vi "Boolean Latch.vi"(1 "Input":bool) -> (0 "Output":bool)   [LabVIEW 2011]
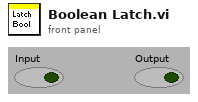
[diagram p1: front panel]
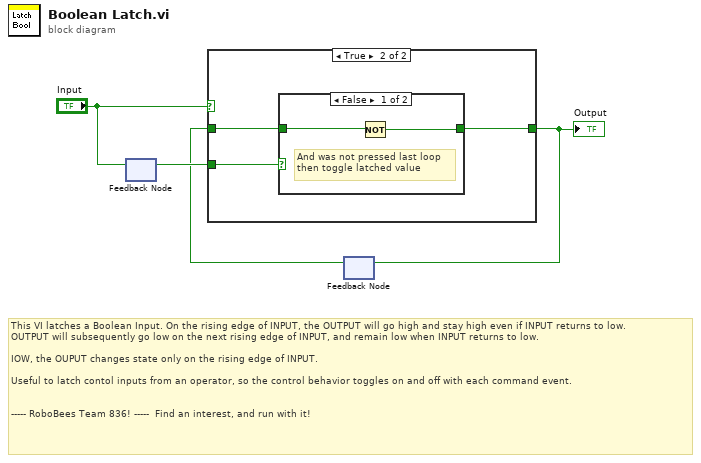
[diagram p0: block diagram]
diagram:
  # "This VI latches a Boolean Input. On the rising edge of INPUT, the OUTPUT will go high and stay high even if INPUT returns to low.\nOUTPUT will subsequently go low on the next rising edge of INPUT, and remain low when INPUT returns to low.\n\nIOW, the OUPUT changes state only on the rising edge of INPUT.\n\nUseful to latch contol inputs from an operator, so the control behavior toggles on and off with each command event. \n\n\n----- RoboBees Team 836! -----  Find an interest, and run with it!"
  n1 = feedback-in #1("Input") -> ()
  n2 = feedback #1() -> (w3:bool)  [unwired: 1 out]
  n3 = feedback #2() -> (w1:bool)  [unwired: 1 out]
  n4 = case shown="True" "Input" {
    tunnel: [w5 w8] -> w2
    tunnel: w3 -> [_ w6]
    tunnel: w1 -> [w5 w7]
    frame False {
      # "If button is not pressed, do nothing"
    }
    frame True {
      n5 = case shown="False" w6 {
        tunnel: [w10 w11] -> w8
        tunnel: w7 -> [w9 w11]
        frame False {
          # "And was not pressed last loop\nthen toggle latched value"
          n6 = Not(x=w9) -> (.not. x?=w10:bool)
        }
        frame True {
          # "And was pressed last loop\nthen hold current latched value"
        }
      }
    }
  }
  "Output" <- w2
  n7 = feedback-in #2(w2) -> ()
